vi "Get Set.vi"(0 "DBSet in":refnum<class "DBSet.lvclass">, 11 "error in (no error)":errorcluster {"code" format="Error %.0f"}) -> (4 "DBSet out":refnum<class "DBSet.lvclass">, 6 "Set":set{string}(c389), 15 "error out":errorcluster {"code" format="Error %.0f"})   [LabVIEW 2020, in "DBSet.lvclass"]
uses:
  DBSet.lvclass
  DBSet.lvclass/DBSet.ctl
  <vilib>/drjdpowell/SQLite Library/SQLite.lvlib
  <vilib>/drjdpowell/SQLite Library/SQL Connection/Execute SQL (1D String).vi
  <vilib>/drjdpowell/SQLite Library/SQL Connection/Connection.lvclass
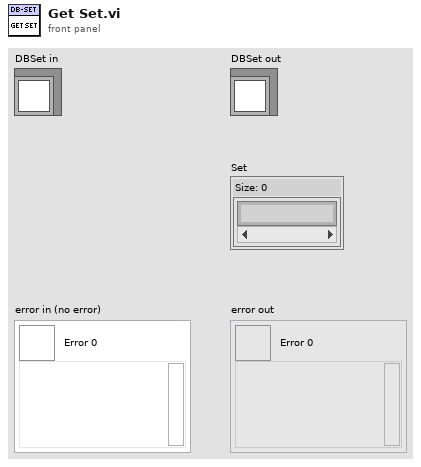
[diagram p1: front panel]
types:
  T1 = typedef "Semaphore RefNum" = refnum<k1>
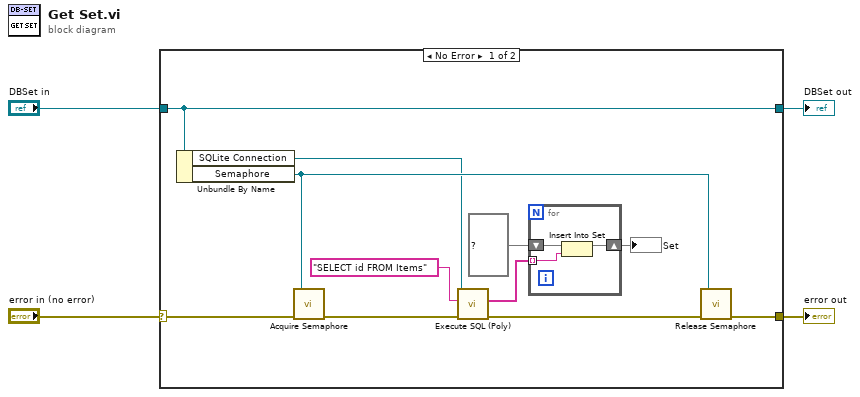
[diagram p0: block diagram]
diagram:
  n1 = case shown="No Error" "error in (no error)" {
    selector: "error in (no error)" -> [w14 w20]
    tunnel: [w13 w20] -> w3
    tunnel: [w15 w19] -> w1
    tunnel: "DBSet in" -> [w15 w19]
    frame No Error {
      n2 = Unbundle By Name(w15) -> ("SQLite Connection"=w6:refnum<class "Connection.lvclass">, "Semaphore"=w12:T1)
      n3 = call <vilib>:"Acquire Semaphore.vi"("error in (no error)"=w14, "semaphore"=w12) -> ("error out"=w8:errorcluster)  [unwired: 3 in, 2 out]
      n4 = call-poly <vilib>:"Execute SQL (Poly).vi"("error in (no error)"=w8, "SQL"="SELECT id FROM Items", "SQLite Connection in"=w6) -> ("error out"=w7:errorcluster, "Result Set"=w10:string[])  [unwired: 5 in, 2 out]
      n5 = for {
        tunnel: w10 -> [w18] mode=indexing
        shift-right: [w16] -> w11
        shift-left: set{string} {} ("Set") -> [w17]
        n6 = Insert Into Set(10:w18, 11:w17) -> (3:w16:set{string})  [unwired: 1 out]
      }
      "Set" <- w11
      n7 = call <vilib>:"Release Semaphore.vi"("error in (no error)"=w7, "semaphore"=w12) -> ("error out"=w13:errorcluster)  [unwired: 4 in, 1 out]
    }
    frame Error {
    }
  }
  "error out" <- w3
  "DBSet out" <- w1
